vi "DataSocketOutput-Daemon.vi"(3 "Configuration":T1, 4 "OutputRequest\nuser event refnum":T2) -> ()   [LabVIEW 2011]
doc: "OutputRequest handler for the DataSocketOutput output device. \n\nThis VI is meant to be started asynchronously. It will register itself as a listener on the OutputRequest user event refnum and process any requests that it knows how to handle.\n\nThe \"Configuration\" structure is used for initialization and contains:\n\"DataSocket URL\": URL of the DataSocket to write to\n\nCommands handled by this VI:\nTarget = \"all\"\n stop: Unregisters and stops running.\nTarget = \"\"timestamp\" or \"timestamped*\"\n [message];* Writes message to DataSocket"
uses:
  Typedefs/OutputRequest refnum.ctl
  Typedefs/OutputRequest.ctl
  DataSocketOutput-Configuration.ctl
panel:
  out "connection id":refnum<k13>
  # "Just a local variable\nfor programming\nconvenience"
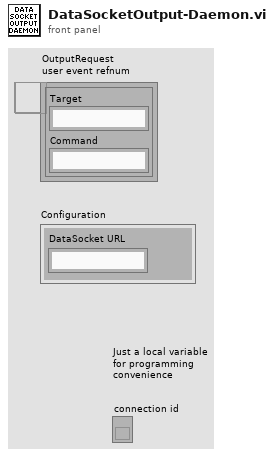
[diagram p1: front panel]
types:
  T1 = typedef "DataSocketOutput-Configuration.ctl" = cluster{"DataSocket URL":string}
  T2 = typedef "OutputRequest refnum.ctl" = refnum<user-event>
  T3 = enum16{"Read", "Write", "ReadWrite", "BufferedRead", "BufferedReadWrite"}
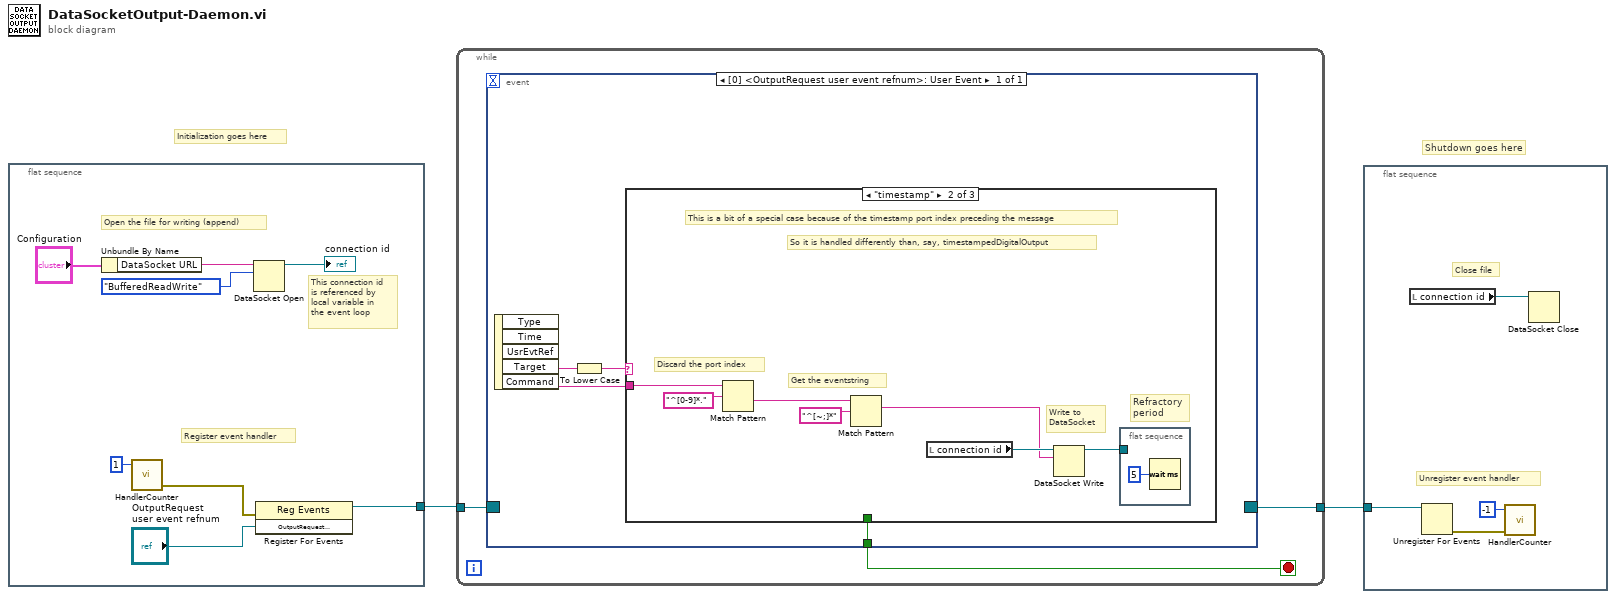
[diagram p0: block diagram]
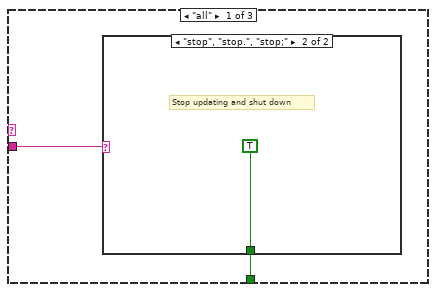
[diagram p2: hidden frame]
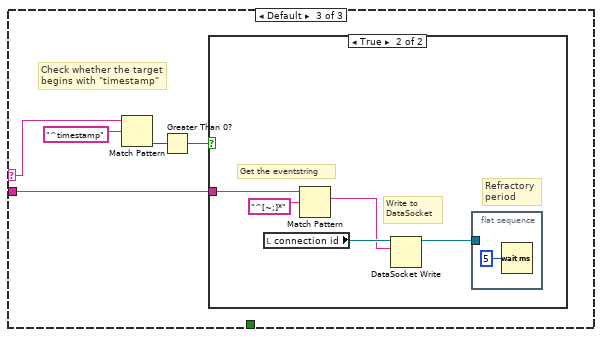
[diagram p4: hidden frame]
diagram:
  # "Shutdown goes here"
  # "Initialization goes here"
  n1 = flat-sequence {
    tunnel: [w10] -> w2
    frame #0 {
      # "Open the file for writing (append)"
      # "This connection id\nis referenced by\nlocal variable in\nthe event loop"
      # "Register event handler"
      n2 = Unbundle By Name("Configuration") -> ("DataSocket URL"=w5:string)
      n3 = call "HandlerCounter.vi"("Change in count"=i16 1) -> ("error out"=w9:errorcluster)  [unwired: 3 in, 1 out]
      n4 = DataSocket Open(10:T3."BufferedReadWrite" ("mode"), 11:w5) -> (3:→"connection id":refnum<k13>)  [unwired: 2 in, 1 out]
      n5 = register-events(error in=w9, "OutputRequest\nuser event refnum") -> (reference out=w10:refnum<event-registration>)  [unwired: 1 in, 1 out]
    }
  }
  n6 = while {
    tunnel: w2 -> [w13]
    tunnel: [w12] -> w1
    stop <- w11 stop-if-true
    n7 = event shown="[0] <OutputRequest\nuser event refnum>: User Event" {
      selector: w13 -> [_]
      dyn-events: [_] -> w12
      timeout: _ -> [_]
      tunnel: [w17] -> w11
      event User Event {
        n8 = event-data() -> ("Target"=w16:string, "Command"=w14:string)  [unwired: 1 in, 3 out]
        n9 = To Lower Case(string=w16) -> (all lower case string=w15:string)
        n10 = case shown="\"timestamp\"" w15 {
          selector: w15 -> [_ _ w32]
          tunnel: w14 -> [w19 w23 w29]
          tunnel: [w18 _ _] -> w17
          frame "all" {
            n11 = case shown="\"stop\", \"stop.\", \"stop;\"" w19 {
              tunnel: [_ TRUE] -> w18
              frame Default {
                # "We should probably put some\nerror throwing code here..."
              }
              frame "stop", "stop.", "stop;" {
                # "Stop updating and shut down"
              }
            }
          }
          frame "timestamp" {
            # "Refractory \nperiod"
            # "Discard the port index"
            # "Get the eventstring"
            # "Write to\nDataSocket"
            # "So it is handled differently than, say, timestampedDigitalOutput"
            # "This is a bit of a special case because of the timestamp port index preceding the message"
            n12 = Match Pattern(string=w23, regular expression="^[0-9]*.") -> (after substring=w24:string)  [unwired: 1 in, 3 out]
            n13 = Match Pattern(string=w24, regular expression="^[~;]*") -> (match substring=w22:string)  [unwired: 1 in, 3 out]
            n14 = local read "connection id"() -> (w26:refnum<k13>)
            n15 = DataSocket Write(10:w22, 11:w26) -> (3:w21:refnum<k13>)  [unwired: 2 in, 2 out]
            n16 = flat-sequence {
              tunnel: w21 -> [_]
              frame #0 {
                n17 = Wait (ms)(milliseconds to wait=u32 5) -> ()  [unwired: 1 out]
              }
            }
          }
          frame Default {
            # "Check whether the target\nbegins with \"timestamp\""
            n18 = Match Pattern(string=w32, regular expression="^timestamp") -> (offset past match=w31:i32)  [unwired: 1 in, 3 out]
            n19 = Greater Than 0?(x=w31) -> (x > 0?=w30:bool)
            n20 = case shown="True" w30 {
              tunnel: w29 -> [_ w37]
              frame False {
                # "Ignore the request, it doesn't pertain\nto this output device"
              }
              frame True {
                # "Refractory \nperiod"
                # "Get the eventstring"
                # "Write to\nDataSocket"
                n21 = local read "connection id"() -> (w38:refnum<k13>)
                n22 = Match Pattern(string=w37, regular expression="^[~;]*") -> (match substring=w35:string)  [unwired: 1 in, 3 out]
                n23 = DataSocket Write(10:w35, 11:w38) -> (3:w34:refnum<k13>)  [unwired: 2 in, 2 out]
                n24 = flat-sequence {
                  tunnel: w34 -> [_]
                  frame #0 {
                    n25 = Wait (ms)(milliseconds to wait=u32 5) -> ()  [unwired: 1 out]
                  }
                }
              }
            }
          }
        }
      }
    }
  }
  n26 = flat-sequence {
    tunnel: w1 -> [w43]
    frame #0 {
      # "Close file"
      # "Unregister event handler"
      n27 = local read "connection id"() -> (w40:refnum<k13>)
      n28 = Unregister For Events(event registration refnum=w43) -> (error out=w42:errorcluster)  [unwired: 1 in]
      n29 = call "HandlerCounter.vi"("error in"=w42, "Change in count"=i16 -1) -> ()  [unwired: 2 in, 2 out]
      n30 = DataSocket Close(11:w40) -> ()  [unwired: 2 in, 2 out]
    }
  }
